vi "FindMatchingSignalNames.vi"(2 "Signal Name":string, 3 "Trigger Data":T3) -> (0 "Anything Found":bool, 1 "Signal Names Matched":string[](array[string]))   [LabVIEW 2016]
uses:
  Ctrl_Signal.ctl
  Ctrl_Signal_Map.ctl
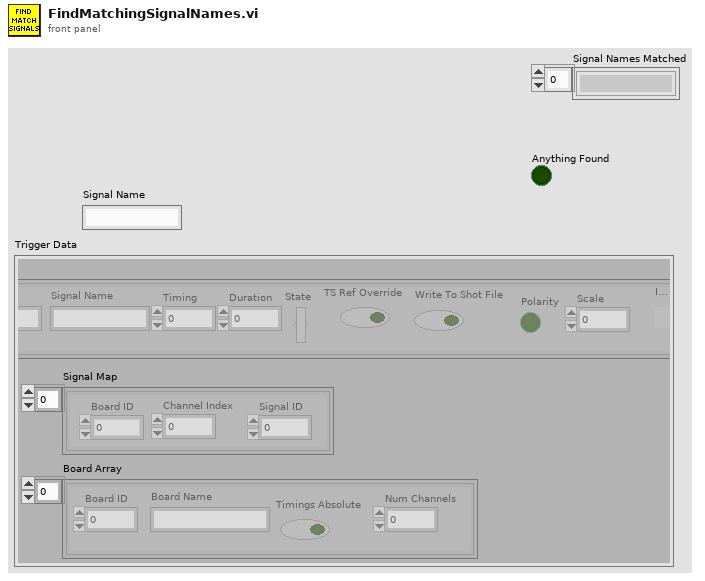
[diagram p1: front panel]
types:
  T1 = typedef "Ctrl_Signal.ctl" = cluster{"Signal Name":string, "Timing":dbl, "Duration":dbl, "State":bool, "TS Ref Override":bool, "Write To Shot File":bool, "Polarity":bool, "Signal ID":dbl, "Scale":dbl, "IsDelay":bool}
  T2 = typedef "Ctrl_Signal_Map.ctl" = cluster{"Channel Index":dbl, "Board ID":dbl, "Signal ID":dbl}
  T3 = cluster{"Signal Array":T1[], "Signal Map":T2[], "Board Array":cluster{"Board ID":dbl, "Board Name":string, "Timings Absolute":bool, "Num Channels":dbl}[]}
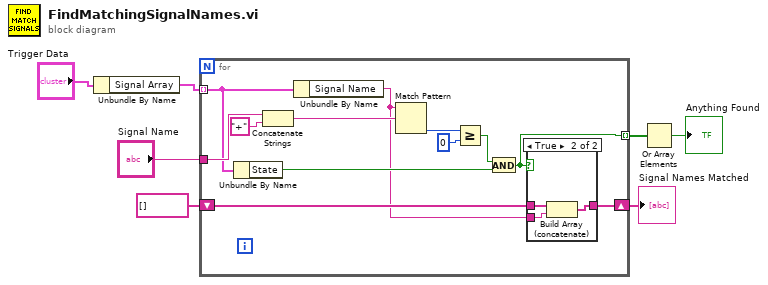
[diagram p0: block diagram]
diagram:
  n1 = Unbundle By Name("Trigger Data") -> ("Signal Array"=w2:T1[])
  n2 = for {
    tunnel: w2 -> [w12] mode=indexing
    tunnel: "Signal Name" -> [w14]
    tunnel: [w9] -> w6 mode=indexing
    shift-right: [w15] -> w1
    shift-left: string[] [] -> [w16]
    n3 = Unbundle By Name(w12) -> ("State"=w10:bool)
    n4 = Concatenate Strings(w14, "+" ("regular expression")) -> (w19:string)
    n5 = Unbundle By Name(w12) -> ("Signal Name"=w8:string)
    n6 = Match Pattern(string=w8, regular expression=w19) -> (offset past match=w18:i32)  [unwired: 1 in, 3 out]
    n7 = Greater Or Equal?(x=w18, y=0) -> (x >= y?=w11:bool)
    n8 = And(x=w11, y=w10) -> (x .and. y?=w9:bool)
    n9 = case shown="True" w9 {
      tunnel: [w20 w23] -> w15
      tunnel: w16 -> [w20 w22]
      tunnel: w8 -> [_ w21]
      frame False {
      }
      frame True {
        n10 = Build Array (concatenate)(w22, w21) -> (w23:string[])
      }
    }
  }
  "Signal Names Matched" <- w1
  n11 = Or Array Elements(Boolean array=w6) -> (logical OR=→"Anything Found":bool)
